vi "Target.vi"() -> ()   [LabVIEW 2018]
uses:
  <vilib>/Platform/TimedLoop/XDataNode/timing_clust.ctl
  <vilib>/Platform/TimedLoop/XDataNode/nitl_modes.ctl
  <vilib>/Platform/TimedLoop/XDataNode/wakeup.ctl
  <vilib>/rvi/eio/common/nirviEmuTemplateMethod_errors.vi
  <vilib>/rvi/Emulation/niFpgaGetClockAttributes.vi
  <vilib>/rvi/Emulation/niFpgaSctlEmulationGetInTimedLoop.vi
  <vilib>/rvi/Emulation/niFpgaEmulationReportErrorSimple.vi
  <vilib>/rvi/Emulation/niFpgaProcessEmulError.vi
  <vilib>/rvi/Emulation/niFpgaCriticalErrorInLSC.vi
  <vilib>/rvi/Memory/Memory_Emulation/niFpgaMemoryFastEmulationDramWriteAndRequestData.vi
  <vilib>/rvi/Memory/Memory_Emulation/niFpgaMemoryEmulationDramWriteAndRequestData.vi
  <vilib>/rvi/DataTransferAndStorage/Container/Common/niFpgaContainerGetUniqueNameForEmu.vi
  <vilib>/rvi/Memory/Memory_Emulation/niFpgaMemoryEmulationDramWriteAndRequestDataApplyByteEnables.vi
  <vilib>/rvi/interface/RandomDataEmulation/niFpgaRandomDataHandleErrors.vi
  <vilib>/eio/EIONode/EIONode.xnode
  <vilib>/Platform/TimedLoop/XDataNode/XDataNode.xnode
  <vilib>/rvi/DataTransferAndStorage/Container/XNode/niFpgaContainer.xnode
  <vilib>/rvi/Memory/Memory_Emulation/niFpgaMemoryEmulationDramRetrieveData.vi
  <vilib>/rvi/interface/RandomDataEmulation/nirviRandomDataFpgaReadWriteTemplate.vi
  <vilib>/Platform/TimedLoop/XDataNode/XDNodeRunTimeDep.lvlib
panel:
  in  "Конец анализа":bool
  in  "Данные":bool
  out "Записали адресов":u32
  in  "-1_прием":i8=-1
  in  "9_прием":i8=9
  out "D1":bool[](array[boolean])
  out "CONTROL":bool[](array[boolean])
  out "D9":bool[](array[boolean])
  in  "SYS_RESET":bool
  in  "Автомат":bool
  in  "FRAME_REQ":bool
  in  "SPI":bool
  out "SPI_OUT":bool[](array[boolean])
  in  "SPI_IN":bool[](array[boolean])=[FALSE, FALSE, FALSE, FALSE, FALSE, FALSE, FALSE, FALSE, FALSE, FALSE, FALSE, FALSE, FALSE, FALSE, FALSE, FALSE]
  out "SPI_OFF":bool
  in  "Нач_адр":u32
  in  "1":u8=1
  in  "2":u8=2
  in  "Кон_адр":u32=16384
  out "Записали FIFO":bool
  in  "REQ_2":u8=7
  in  "REQ_1":u8=2
  in  "Кадр на ПК":bool
  in  "Стоп":bool
  # "R/W"
  # "D0"
  # "A6"
  # "A0"
  # "D7"
  # "D7"
  # "D0"
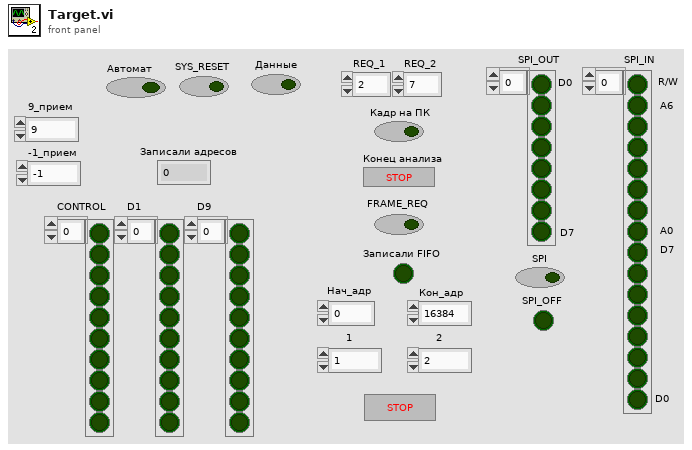
[diagram p1: front panel]
types:
  T1 = typedef "XDNodeRunTimeDep.lvlib/timing_clust.ctl" = cluster{"Expected End [f-1]":u64, "Actual End [f-1]":u64, "Finished Late? [f-1]":bool, "Expected End [i-1]":u64, "Actual End [i-1]":u64, "Finished Late? [i-1]":bool, "Expected Start [i]":u64, "Actual Start [i]":u64, "Expected Start [f]":u64, "Actual Start [f]":u64, "Source Name":string, "Structure Name":string, "Period":i64, "Deadline":i64, "Offset":i64, "Start":i64, "Priority":i32, "Timeout":i32, "Mode":T2, "Wakeup Reason":T3, "Error":errorcluster, "Source Type":string, "Secondary Source Type":string, "Global End Time":u64, "Global Start Time":u64, "Frame Duration":u64, "Iteration Duration":u64, "Assigned CPU":i32, "I/O Scan Engine Mode":u32}
  T2 = typedef "XDNodeRunTimeDep.lvlib/nitl_modes.ctl" = enum32{"No Change", "Process missed periods, maintain original phase", "Discard missed periods, maintain original phase", "Process missed periods, ignore original phase", "Discard missed periods, ignore original phase"}
  T3 = typedef "XDNodeRunTimeDep.lvlib/wakeup.ctl" = enum32{"Normal", "Aborted", "Asynchronous wakeup", "Timing source error", "Timed loop error", "Timeout"}
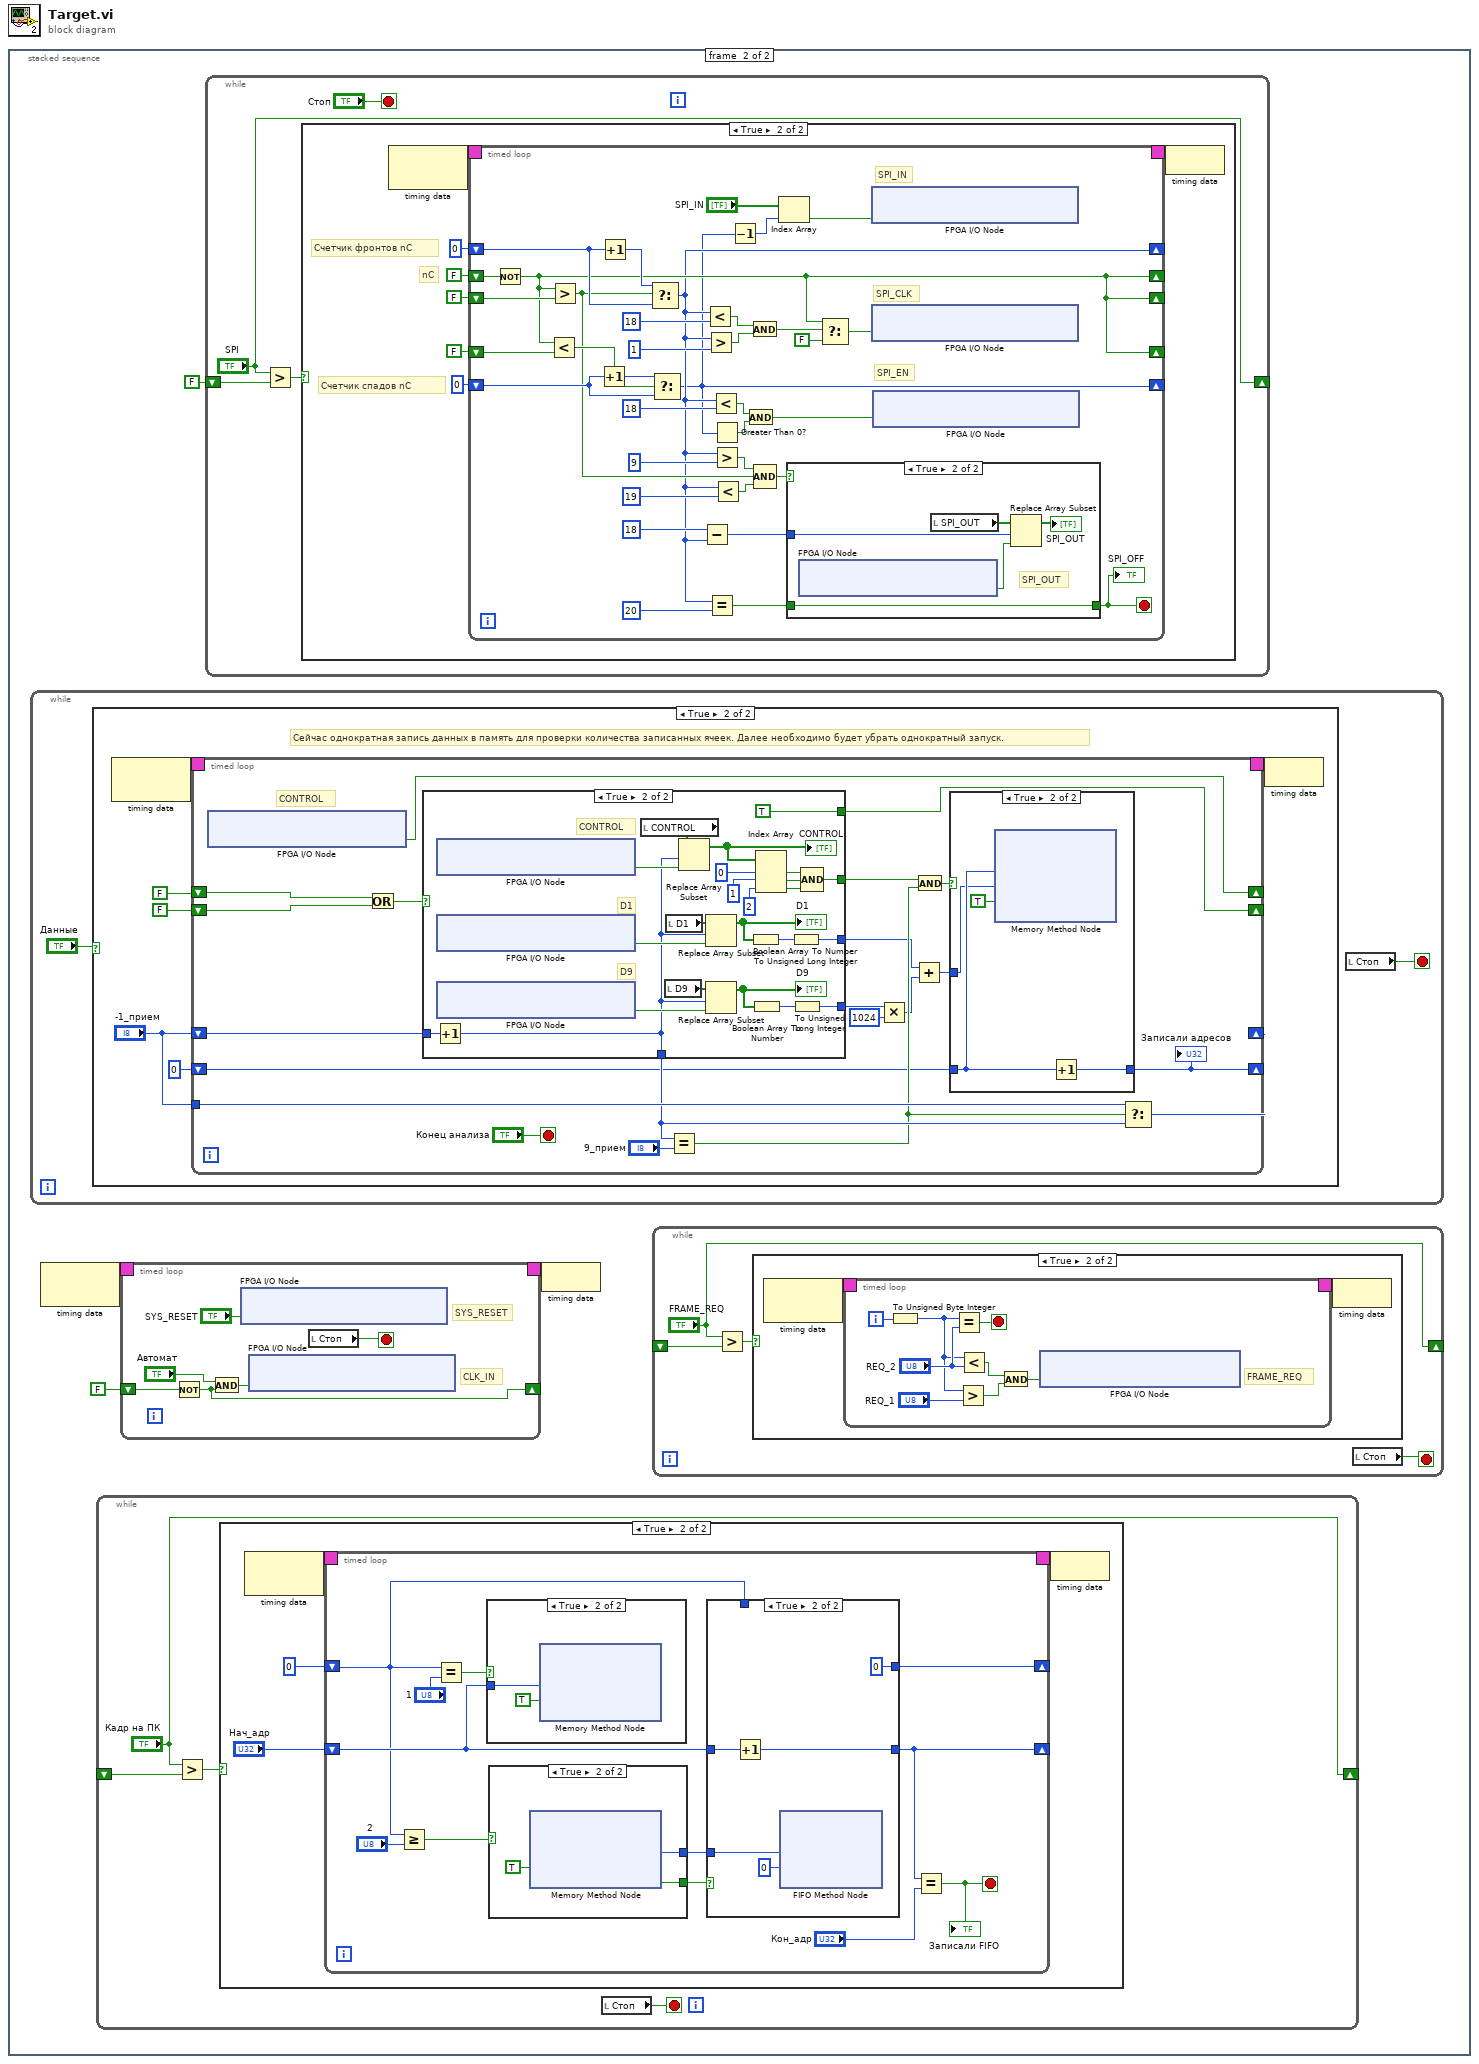
[diagram p0: block diagram]
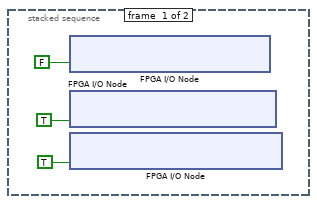
[diagram p2: hidden frame]
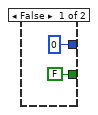
[diagram p5: hidden frame]
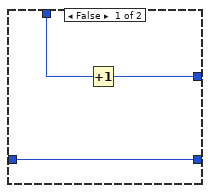
[diagram p7: hidden frame]
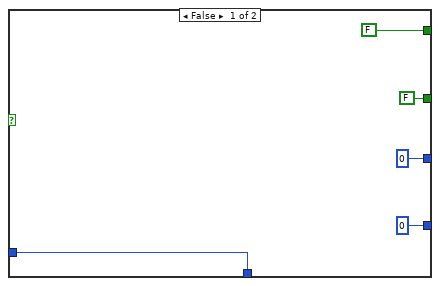
[diagram p10: hidden frame]
diagram:
  n1 = stacked-sequence {
    frame #0 {
      n2 = xnode "FPGA I/O Node"("IO Module\\DDCA_DIO0-7_WE"=FALSE ("IO Module\\DDCA_DIO0-7_WE")) -> ()  [unwired: 1 in, 1 out]
      n3 = xnode "FPGA I/O Node"("IO Module\\DDCA_DIO8-15_WE"=TRUE ("IO Module\\DDCA_DIO8-15_WE")) -> ()  [unwired: 1 in, 1 out]
      n4 = xnode "FPGA I/O Node"("IO Module\\DDCA_DIO16-23_WE"=TRUE ("IO Module\\DDCA_DIO16-23_WE")) -> ()  [unwired: 1 in, 1 out]
    }
    frame #1 {
      n5 = while {
        stop <- w65 stop-if-true
        n6 = case shown="True" "Данные" {
          frame False {
          }
          frame True {
            # "Сейчас однократная запись данных в память для проверки количества записанных ячеек. Далее необходимо будет убрать однократный запуск."
            n7 = node-c288() -> (w72:T1)  [unwired: 1 in]
            n8 = timed-loop {
              timing: w72 -> [_]
              timing-out: [_] -> w71
              shift-right: [w87] -> _
              shift-left: "-1_прием" -> [w93]
              shift-right: [w92] -> _
              shift-left: FALSE -> [w89]
              shift-right: [w88] -> _
              shift-left: FALSE -> [w90]
              tunnel: "-1_прием" -> [w85]
              shift-right: [w75] -> _
              shift-left: u32 0 -> [w81]
              stop <- "Конец анализа" stop-if-true
              # "CONTROL"
              n9 = xnode "FPGA I/O Node"() -> ("IO Module\\DDCA_DIO4_Read"=w92:bool)  [unwired: 1 in, 1 out]
              n10 = Or(x=w89, y=w90) -> (x .or. y?=w91:bool)
              n11 = case shown="True" w91 {
                tunnel: w93 -> [w102 w121]
                tunnel: [FALSE TRUE] -> w88
                tunnel: [w102 w118] -> w84
                tunnel: [u16 0 w106] -> w77
                tunnel: [u16 0 w105] -> w80
                tunnel: [FALSE w108] -> w73
                frame False {
                }
                frame True {
                  # "CONTROL"
                  # "D9"
                  # "D1"
                  n12 = Increment(x=w121) -> (x+1=w118:i8)
                  n13 = xnode "FPGA I/O Node"() -> ("IO Module\\DDCA_DIO4_Read"=w119:bool)  [unwired: 1 in, 1 out]
                  n14 = xnode "FPGA I/O Node"() -> ("IO Module\\DDCA_DIO1_Read"=w123:bool)  [unwired: 1 in, 1 out]
                  n15 = xnode "FPGA I/O Node"() -> ("IO Module\\DDCA_DIO0_Read"=w122:bool)  [unwired: 1 in, 1 out]
                  n16 = local read "CONTROL"() -> (w126:bool[])
                  n17 = local read "D9"() -> (w124:bool[])
                  n18 = local read "D1"() -> (w125:bool[])
                  n19 = Replace Array Subset(array=w126, new element=w119, index=w118) -> (w115:bool[])
                  "CONTROL" <- w115
                  n20 = Replace Array Subset(array=w125, new element=w123, index=w118) -> (w117:bool[])
                  "D1" <- w117
                  n21 = Replace Array Subset(array=w124, new element=w122, index=w118) -> (w116:bool[])
                  "D9" <- w116
                  n22 = Boolean Array To Number(Boolean array=w117) -> (number=w107:u16)
                  n23 = Boolean Array To Number(Boolean array=w116) -> (number=w104:u16)
                  n24 = Index Array(array=w115, index #1=0 ("index"), index #2=1 ("index"), index #3=2 ("index")) -> (element #1=w111:bool, element #2=w110:bool, element #3=w109:bool)
                  n25 = To Unsigned Long Integer(number=w107) -> (unsigned 32bit integer=w106:u32)
                  n26 = To Unsigned Long Integer(number=w104) -> (unsigned 32bit integer=w105:u32)
                  n27 = Compound Arithmetic op=AND(w111, w110, w109) -> (w108:bool)
                }
              }
              n28 = Equal?(x=w84, y="9_прием") -> (x = y?=w83:bool)
              n29 = Multiply(x=w80, y=u32 1024) -> (x*y=w78:u32)
              n30 = Add(x=w77, y=w78) -> (x+y=w76:u32)
              n31 = And(x=w73, y=w83) -> (x .and. y?=w82:bool)
              n32 = case shown="True" w82 {
                tunnel: w81 -> [w94 w98]
                tunnel: [w94 w97] -> w75
                tunnel: w76 -> [_ w96]
                frame False {
                }
                frame True {
                  n33 = xnode ("Memory Method Node")("Address"=w98, "Data"=w96, "Input Valid"=TRUE) -> ()  [unwired: 1 in, 2 out]
                  n34 = Increment(x=w98) -> (x+1=w97:u32)
                }
              }
              "Записали адресов" <- w75
              n35 = Select(t=w85, s=w83, f=w84) -> (s? t:f=w87:i8)
            }
            n36 = node-c288(w71) -> ()
          }
        }
        n37 = local read "Стоп"() -> (w65:bool)
      }
      n38 = node-c288() -> (w7:T1)  [unwired: 1 in]
      n39 = while {
        shift-right: ["Кадр на ПК"] -> _
        shift-left: _ -> [w27]
        stop <- w29 stop-if-true
        n40 = Greater?(x="Кадр на ПК", y=w27) -> (0:w28:bool)
        n41 = case shown="True" w28 {
          frame False {
          }
          frame True {
            n42 = node-c288() -> (w33:T1)  [unwired: 1 in]
            n43 = timed-loop {
              shift-right: [w44] -> _
              shift-left: "Нач_адр" -> [w38]
              timing: w33 -> [_]
              timing-out: [_] -> w32
              shift-right: [w35] -> _
              shift-left: u8 0 -> [w36]
              stop <- w45 stop-if-true
              n44 = Greater Or Equal?(x=w36, y="2") -> (x >= y?=w39:bool)
              n45 = Equal?(x=w36, y="1") -> (x = y?=w42:bool)
              n46 = case shown="True" w42 {
                tunnel: w38 -> [_ w51]
                frame False {
                }
                frame True {
                  n47 = xnode ("Memory Method Node")("Address"=w51, "Input Valid"=TRUE) -> ()  [unwired: 1 in, 2 out]
                }
              }
              n48 = case shown="True" w39 {
                tunnel: [u8 0 ("Data") w49] -> w43
                tunnel: [FALSE ("Output Valid") w48] -> w37
                frame False {
                }
                frame True {
                  n49 = xnode ("Memory Method Node")("Ready for Output"=TRUE ("Ready For Output")) -> ("Data"=w49:u32, "Output Valid"=w48:bool)  [unwired: 1 in, 1 out]
                }
              }
              n50 = case shown="True" w37 {
                tunnel: [w53 w60] -> w44
                tunnel: w43 -> [_ w56]
                tunnel: w38 -> [w53 w59]
                tunnel: w36 -> [w55 _]
                tunnel: [w54 u8 0] -> w35
                frame False {
                  n51 = Increment(x=w55) -> (x+1=w54:u8)
                }
                frame True {
                  n52 = Increment(x=w59) -> (x+1=w60:u32)
                  n53 = xnode ("FIFO Method Node")("Element"=w56, "Timeout"=0) -> ()  [unwired: 1 in, 2 out]
                }
              }
              n54 = Equal?(x=w44, y="Кон_адр") -> (x = y?=w45:bool)
              "Записали FIFO" <- w45
            }
            n55 = node-c288(w32) -> ()
          }
        }
        n56 = local read "Стоп"() -> (w29:bool)
      }
      n57 = timed-loop {
        timing: w7 -> [_]
        timing-out: [_] -> w6
        shift-right: [w133] -> _
        shift-left: FALSE -> [w136]
        stop <- w131 stop-if-true
        # "SYS_RESET"
        # "CLK_IN"
        n58 = Not(x=w136) -> (.not. x?=w133:bool)
        n59 = And(x="Автомат", y=w133) -> (x .and. y?=w134:bool)
        n60 = xnode "FPGA I/O Node"("IO Module\\DDCA_DIO17_Write"="SYS_RESET") -> ()  [unwired: 1 in, 1 out]
        n61 = xnode "FPGA I/O Node"("IO Module\\DDCA_DIO18_Write"=w134) -> ()  [unwired: 1 in, 1 out]
        n62 = local read "Стоп"() -> (w131:bool)
      }
      n63 = while {
        shift-right: ["SPI"] -> _
        shift-left: FALSE ("SPI") -> [w142]
        stop <- "Стоп" stop-if-true
        n64 = Greater?(x="SPI", y=w142) -> (0:w143:bool)
        n65 = case shown="True" w143 {
          frame False {
          }
          frame True {
            # "Счетчик спадов nC"
            # "nC"
            # "Счетчик фронтов nC"
            n66 = node-c288() -> (w151:T1)  [unwired: 1 in]
            n67 = timed-loop {
              timing: w151 -> [_]
              timing-out: [_] -> w150
              shift-right: [w165] -> _
              shift-left: FALSE -> [w187]
              shift-right: [w165] -> _
              shift-left: FALSE -> [w186]
              shift-right: [w154] -> _
              shift-left: u8 0 -> [w185]
              shift-right: [w165] -> _
              shift-left: FALSE -> [w184]
              shift-right: [w152] -> _
              shift-left: u8 0 -> [w181]
              stop <- w169 stop-if-true
              # "SPI_IN"
              # "SPI_EN"
              # "SPI_CLK"
              n68 = Not(x=w187) -> (.not. x?=w165:bool)
              n69 = Less?(x=w165, y=w184) -> (x < y?=w183:bool)
              n70 = Greater?(x=w165, y=w186) -> (0:w166:bool)
              n71 = Increment(x=w181) -> (x+1=w182:u8)
              n72 = Increment(x=w185) -> (x+1=w172:u8)
              n73 = Select(t=w172, s=w166, f=w185) -> (s? t:f=w154:u8)
              n74 = Select(t=w182, s=w183, f=w181) -> (s? t:f=w152:u8)
              n75 = Subtract(x=u8 18 ("17_READ"), y=w154) -> (x-y=w153:u8)
              n76 = Less?(x=w154, y=u8 18 ("18_CLK")) -> (x < y?=w163:bool)
              n77 = Greater?(x=w154, y=u8 1 ("1")) -> (0:w162:bool)
              n78 = Equal?(x=w154, y=u8 20 ("19_20")) -> (x = y?=w170:bool)
              n79 = Less?(x=w154, y=u8 18 ("18_EN")) -> (x < y?=w176:bool)
              n80 = Greater Than 0?(x=w152) -> (x > 0?=w177:bool)
              n81 = Greater?(x=w154, y=u8 9 ("9")) -> (0:w167:bool)
              n82 = Less?(x=w154, y=u8 19 ("18_READ")) -> (x < y?=w157:bool)
              n83 = Decrement(x=w152) -> (x-1=w173:u8)
              n84 = And(x=w176, y=w177) -> (x .and. y?=w175:bool)
              n85 = And(x=w163, y=w162) -> (x .and. y?=w179:bool)
              n86 = Compound Arithmetic op=AND(w167, w166, w157) -> (w168:bool)
              n87 = Index Array(array="SPI_IN", index=w173) -> (element=w171:bool)
              n88 = case shown="True" w168 {
                tunnel: [w188 w190] -> w169
                tunnel: w170 -> [w188 w190]
                tunnel: w153 -> [_ w189]
                frame False {
                }
                frame True {
                  # "SPI_OUT"
                  n89 = xnode "FPGA I/O Node"() -> ("IO Module\\DDCA_DIO7_Read"=w191:bool)  [unwired: 1 in, 1 out]
                  n90 = local read "SPI_OUT"() -> (w192:bool[])
                  n91 = Replace Array Subset(array=w192, new element=w191, index=w189) -> (→"SPI_OUT":bool[])
                }
              }
              "SPI_OFF" <- w169
              n92 = Select(t=w165, s=w179, f=FALSE) -> (s? t:f=w178:bool)
              n93 = xnode "FPGA I/O Node"("IO Module\\DDCA_DIO14_Write"=w171) -> ()  [unwired: 1 in, 1 out]
              n94 = xnode "FPGA I/O Node"("IO Module\\DDCA_DIO16_Write"=w178) -> ()  [unwired: 1 in, 1 out]
              n95 = xnode "FPGA I/O Node"("IO Module\\DDCA_DIO15_Write"=w175) -> ()  [unwired: 1 in, 1 out]
            }
            n96 = node-c288(w150) -> ()
          }
        }
      }
      n97 = node-c288(w6) -> ()
      n98 = while {
        shift-right: ["FRAME_REQ"] -> _
        shift-left: _ -> [w10]
        stop <- w8 stop-if-true
        n99 = Greater?(x="FRAME_REQ", y=w10) -> (0:w11:bool)
        n100 = case shown="True" w11 {
          frame False {
          }
          frame True {
            n101 = node-c288() -> (w13:T1)  [unwired: 1 in]
            n102 = timed-loop {
              timing: w13 -> [_]
              timing-out: [_] -> w12
              i -> [w15]
              stop <- w18 stop-if-true
              # "FRAME_REQ"
              n103 = To Unsigned Byte Integer(number=w15) -> (unsigned 8bit integer=w14:u8)
              n104 = Equal?(x=w14, y="REQ_2") -> (x = y?=w18:bool)
              n105 = Greater?(x=w14, y="REQ_1") -> (0:w20:bool)
              n106 = Less?(x=w14, y="REQ_2") -> (x < y?=w21:bool)
              n107 = And(x=w21, y=w20) -> (x .and. y?=w17:bool)
              n108 = xnode "FPGA I/O Node"("IO Module\\DDCA_DIO8_Write"=w17) -> ()  [unwired: 1 in, 1 out]
            }
            n109 = node-c288(w12) -> ()
          }
        }
        n110 = local read "Стоп"() -> (w8:bool)
      }
    }
  }
